vi "RGSBias_Wrapper.vi"(0 "Path Array":string[](array[string]), 1 "Input Values":dbl[](array[numeric])) -> ()   [LabVIEW 2018]
uses:
  <vilib>/Analysis/1siggen.llb/Ramp Pattern by Samples.vi
  <vilib>/DAQmx/write.llb/DAQmx Write (Analog 1D DBL 1Chan NSamp).vi
  <vilib>/DAQmx/create/channels.llb/DAQmx Create Channel (AO-Voltage-Basic).vi
  <vilib>/DAQmx/configure/timing.llb/DAQmx Timing (Sample Clock).vi
  <vilib>/DAQmx/miscellaneous.llb/DAQmx Fill In Error Info.vi
  <vilib>/Analysis/NI_AALBase.lvlib
panel:
  out "Output Value":dbl
  out "pathName":path
  out "Device":string
  in  "rate":dbl=1000.0 format="%0.2f"
  in  "samples":i32=128
  out "Start Value":dbl
  out "End Value":dbl
  out "Enable RGS Bias?":bool
  out "Time (s)":dbl
  out "Device names":string[](array[string])=[" Dev5/ao4", "", "", "", ""]
  out "Initial Val, Gain":dbl[](array[numeric])=[119.0, 161.0, -0.006, 0.0]
  out "error out":errorcluster
  # "RGS Bias Dev5/ao4"
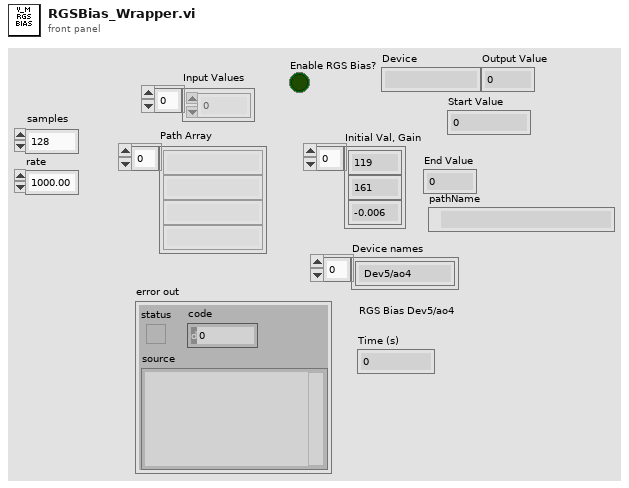
[diagram p1: front panel]
types:
  T1 = enum16{"open", "replace", "create", "open or create", "replace or create", "replace or create with confirmation"}
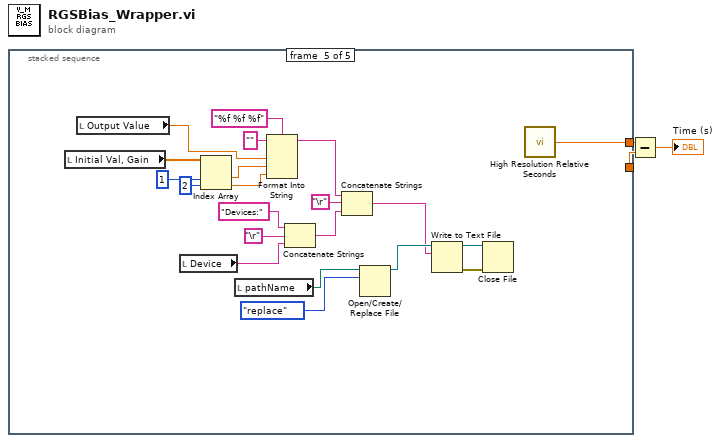
[diagram p0: block diagram]
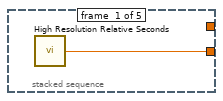
[diagram p2: hidden frame]
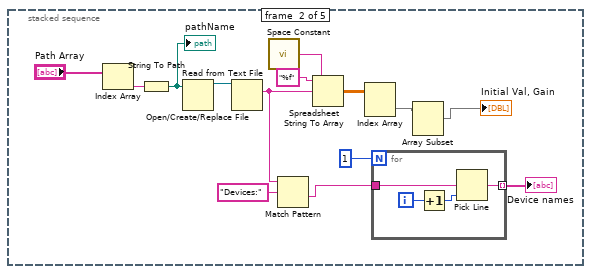
[diagram p3: hidden frame]
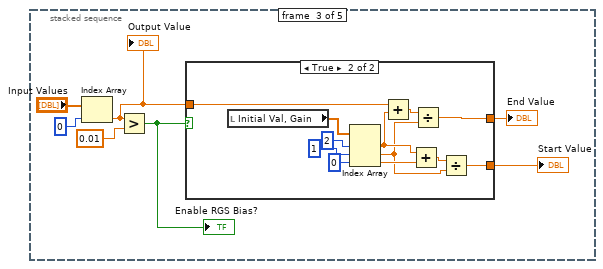
[diagram p4: hidden frame]
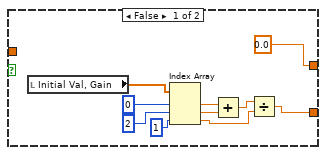
[diagram p5: hidden frame]
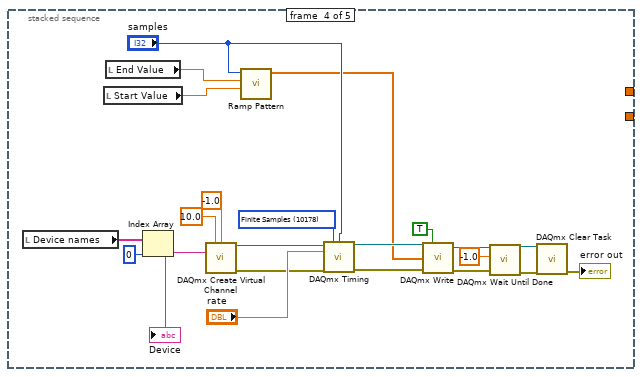
[diagram p6: hidden frame]
diagram:
  n1 = stacked-sequence {
    tunnel: [w4 _ _ _ _] -> w2
    tunnel: [_ _ _ _ w94] -> w3
    frame #0 {
      n2 = call <vilib>:"High Resolution Relative Seconds.vi"() -> ("relative seconds"=w4:dbl)
    }
    frame #1 {
      n3 = Index Array(array="Path Array") -> (element=w17:string)  [unwired: 1 in]
      n4 = String To Path(string=w17) -> (path=w7:path)
      "pathName" <- w7
      n5 = Open/Create/Replace File(file path (use dialog)=w7) -> (refnum out=w8:refnum<file>)  [unwired: 5 in, 2 out]
      n6 = Read from Text File(file (use dialog)=w8) -> (text=w13:string)  [unwired: 3 in, 3 out]
      n7 = call <vilib>:"Space Constant.vi"() -> ("String"=w15:string)
      n8 = Match Pattern(string=w13, regular expression="Devices:") -> (after substring=w11:string)  [unwired: 1 in, 3 out]
      n9 = Spreadsheet String To Array(delimiter (Tab)=w15, format string="%f", spreadsheet string=w13) -> (array=w14:dbl[][])  [unwired: 1 in]
      n10 = Index Array(array=w14) -> (element=w6:dbl[])  [unwired: 2 in]
      n11 = for {
        N: 1 -> [_]
        tunnel: w11 -> [w20]
        tunnel: [w19] -> w9 mode=indexing
        i -> [w22]
        n12 = Increment(x=w22) -> (x+1=w21:i32)
        n13 = Pick Line(multi-line string=w20, line index=w21) -> (output string=w19:string)  [unwired: 1 in]
      }
      "Device names" <- w9
      n14 = Array Subset(array=w6) -> (→"Initial Val, Gain":dbl[])  [unwired: 2 in]
    }
    frame #2 {
      n15 = Index Array(array="Input Values", index=0) -> (element=w24:dbl)
      "Output Value" <- w24
      n16 = Greater?(x=w24, y=0.01) -> (0:w27:bool)
      "Enable RGS Bias?" <- w27
      n17 = case shown="True" w27 {
        tunnel: [0.0 w47] -> w26
        tunnel: w24 -> [_ w46]
        tunnel: [w35 w43] -> w23
        frame False {
          n18 = local read "Initial Val, Gain"() -> (w37:dbl[])
          n19 = Index Array(array=w37, index #1=0 ("index"), index #2=2 ("index"), index #3=1 ("index")) -> (element #1=w32:dbl, element #2=w31:dbl, element #3=w30:dbl)
          n20 = Add(x=w32, y=w31) -> (x+y=w38:dbl)
          n21 = Divide(x=w38, y=w30) -> (x/y=w35:dbl)
        }
        frame True {
          n22 = local read "Initial Val, Gain"() -> (w50:dbl[])
          n23 = Index Array(array=w50, index #1=2 ("index"), index #2=1 ("index"), index #3=0 ("index")) -> (element #1=w41:dbl, element #2=w40:dbl, element #3=w42:dbl)
          n24 = Add(x=w46, y=w41) -> (x+y=w51:dbl)
          n25 = Add(x=w41, y=w42) -> (x+y=w44:dbl)
          n26 = Divide(x=w51, y=w40) -> (x/y=w47:dbl)
          n27 = Divide(x=w44, y=w40) -> (x/y=w43:dbl)
        }
      }
      "End Value" <- w26
      "Start Value" <- w23
    }
    frame #3 {
      w60 = 10178 items=["Finite Samples"=10178, "Continuous Samples"=10123, "Hardware Timed Single Point"=12522] ("sample mode")
      n28 = local read "Device names"() -> (w70:string[])
      n29 = local read "Start Value"() -> (w66:dbl)
      n30 = local read "End Value"() -> (w67:dbl)
      n31 = Index Array(array=w70, index=0) -> (element=w68:string)
      "Device" <- w68
      n32 = call-poly <vilib>:"DAQmx Create Virtual Channel.vi"("maximum value"=10.0, "minimum value"=-1.0, "physical channels"=w68) -> ("task out"=w65:refnum<k21>, "error out"=w63:errorcluster)  [unwired: 11 in]
      n33 = call-poly <vilib>:"Ramp Pattern.vi"("start"=w66, "end"=w67, "samples"="samples") -> ("Ramp Pattern"=w58:dbl[])  [unwired: 7 in, 1 out]
      n34 = call-poly <vilib>:"DAQmx Timing.vi"("task/channels in"=w65, "sample mode"=w60, "samples per channel"="samples", "rate"="rate", "error in"=w63) -> ("task out"=w62:refnum<k21>, "error out"=w61:errorcluster)  [unwired: 9 in]
      n35 = call-poly <vilib>:"DAQmx Write.vi"("task/channels in"=w62, "auto start"=TRUE, "data"=w58, "error in"=w61) -> ("task out"=w54:refnum<k21>, "error out"=w53:errorcluster)  [unwired: 9 in, 1 out]
      n36 = call <vilib>:"DAQmx Wait Until Done.vi"("task/channels in"=w54, "timeout (sec)"=-1.0, "error in"=w53) -> ("task out"=w55:refnum<k21>, "error out"=w56:errorcluster)  [unwired: 11 in]
      n37 = call <vilib>:"DAQmx Clear Task.vi"("task in"=w55, "error in"=w56) -> ("error out"=→"error out":errorcluster)  [unwired: 13 in]
    }
    frame #4 {
      n38 = local read "Initial Val, Gain"() -> (w92:dbl[])
      n39 = local read "Output Value"() -> (w87:dbl)
      n40 = local read "Device"() -> (w80:string)
      n41 = Index Array(array=w92, index #1=1 ("index"), index #2=2 ("index")) -> (element #1=w89:dbl, element #2=w88:dbl)
      n42 = local read "pathName"() -> (w79:path)
      n43 = Format Into String(format string="%f %f %f", initial string="", w87, w89, w88) -> (resulting string=w84:string)  [unwired: 1 in, 1 out]
      n44 = Concatenate Strings("Devices:" ("string"), "\r", w80) -> (w83:string)
      n45 = Concatenate Strings(w84, "\r", w83) -> (w76:string)
      n46 = Open/Create/Replace File(file path (use dialog)=w79, operation (0:open)=T1."replace") -> (refnum out=w77:refnum<file>)  [unwired: 4 in, 2 out]
      n47 = Write to Text File(file (use dialog)=w77, text=w76) -> (refnum out=w74:refnum<file>, error out=w75:errorcluster)  [unwired: 2 in, 1 out]
      n48 = Close File(refnum=w74, error in=w75) -> ()  [unwired: 2 out]
      n49 = call <vilib>:"High Resolution Relative Seconds.vi"() -> ("relative seconds"=w94:dbl)
    }
  }
  n50 = Subtract(x=w3, y=w2) -> (x-y=→"Time (s)":dbl)
